vi "Launcher.vi"() -> ()   [LabVIEW 2022 SP3]
uses:
  UDP Input.ctl
  Vision Receiver/Vision Receiver/Vision Receiver.lvclass
  C:/Program Files (x86)/National Instruments/LabVIEW 2022/vi.lib/ActorFramework/Actor/Actor.lvclass
  Vision Receiver/Vision Receiver Messages/Request Msg/Request Msg.lvclass/Request Msg.ctl
  <vilib>/ActorFramework/Message Enqueuer/Message Enqueuer.lvclass/Message Enqueuer.ctl
  <vilib>/ActorFramework/Message Enqueuer/Enqueue.vi
  Vision Receiver/Vision Receiver Messages/Request Msg/Request Msg.lvclass
  C:/Program Files (x86)/National Instruments/LabVIEW 2022/vi.lib/ActorFramework/Message/Message.lvclass
  <vilib>/ActorFramework/Message Priority Queue/Priority Enqueue.vi
  <vilib>/ActorFramework/Actor/Actor.lvclass
  C:/Program Files (x86)/National Instruments/LabVIEW 2022/vi.lib/MGI/Monitored Actor/Monitored Actor/Monitored Actor/Monitored Actor.lvclass
  C:/Users/ebert/Documents/codes/ssl/repo/teste/Vision Receiver/Vision Receiver/Vision Receiver.lvclass
  C:/Users/ebert/Documents/codes/ssl/repo/teste/UDP Data Receiver/UDP Data Receiver/UDP Data Receiver.lvclass
panel:
  in  "stop":bool
  in  "Input":T1={"Local IP"="", "Port"="10020", "Server IP"="224.5.23.2"}
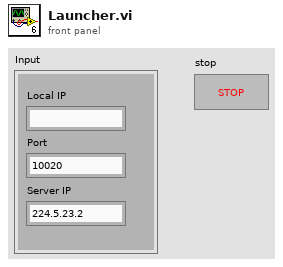
[diagram p1: front panel]
types:
  T1 = typedef "UDP Input.ctl" = cluster{"Local IP":string, "Port":string, "Server IP":string}
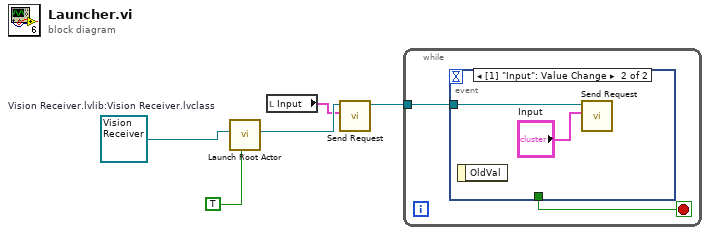
[diagram p0: block diagram]
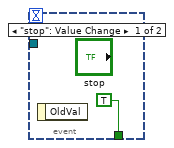
[diagram p2: hidden frame]
diagram:
  w5 = refnum<class "Vision Receiver.lvclass"> refnum  # Vision Receiver.lvlib:Vision Receiver.lvclass
  n1 = call <vilib>:"Launch Root Actor.vi"("Open Actor Core front panel? (F)"=TRUE, "Actor"=w5) -> ("Actor's Enqueuer"=w2:refnum<class "Message Enqueuer.lvclass">)  [unwired: 8 in, 1 out]
  n2 = local read "Input"() -> (w1:T1)
  n3 = call "Send Request.vi"("Input"=w1, "Message Enqueuer in"=w2) -> ("Message Enqueuer out"=w3:refnum<class "Message Enqueuer.lvclass">)  [unwired: 8 in, 1 out]
  n4 = while {
    tunnel: w3 -> [w6]
    stop <- w7 stop-if-true
    n5 = event shown="[1] \"Input\": Value Change" {
      selector: _ -> [_ _]
      dyn-events: _ -> [_ _]
      timeout: _ -> [_ _]
      tunnel: [TRUE _] -> w7
      tunnel: w6 -> [_ w10]
      event "stop": Value Change {
        n6 = event-data() -> ()  [unwired: 1 in, 1 out]
      }
      event Value Change {
        n7 = event-data() -> ()  [unwired: 1 in, 1 out]
        n8 = call "Send Request.vi"("Input"="Input", "Message Enqueuer in"=w10) -> ()  [unwired: 8 in, 2 out]
      }
    }
  }
